vi "joystick-velout.vi"() -> (0 "error out 3":errorcluster, 2 "channel":T1)   [LabVIEW 2016]
uses:
  <extravilib>/ChannelInstances/Lossy Stream-a[.](dbl)/)Channel.ctl
  <extravilib>/ChannelInstances/Lossy Stream-a[.](dbl)/Write With Abort.vi
  <extravilib>/ChannelInstances/Lossy Stream-a[.](dbl)/Endpoint.vi
  <extravilib>/ChannelInstances/Lossy Stream-a[.](dbl)/)Channel.vi
  <resource>/ChannelSupport/_ChannelSupport/WaitIfNeeded.vi
  <vilib>/Utility/inputDevices.llb/closeJoystick.vi
  <extravilib>/ChannelInstances/Lossy Stream-a[.](dbl).lvlib
panel:
  out "16bit integer 3":i16
  out "16bit integer 2":i16
  out "16bit integer":i16
  out "appended array":u8[](array[numeric])
  in  "stop":bool
  in  "pos 1":i16=3468
  in  "pos 2":i16=3468
  in  "pos 3":i16=3468
  out "vel radial":u8[](array[numeric])
  out "vel normal":u8[](array[numeric])
  out "vel rotation":u8[](array[numeric])
  out "drible":u8
  # "vtan"
  # "vnorm"
  # "vang"
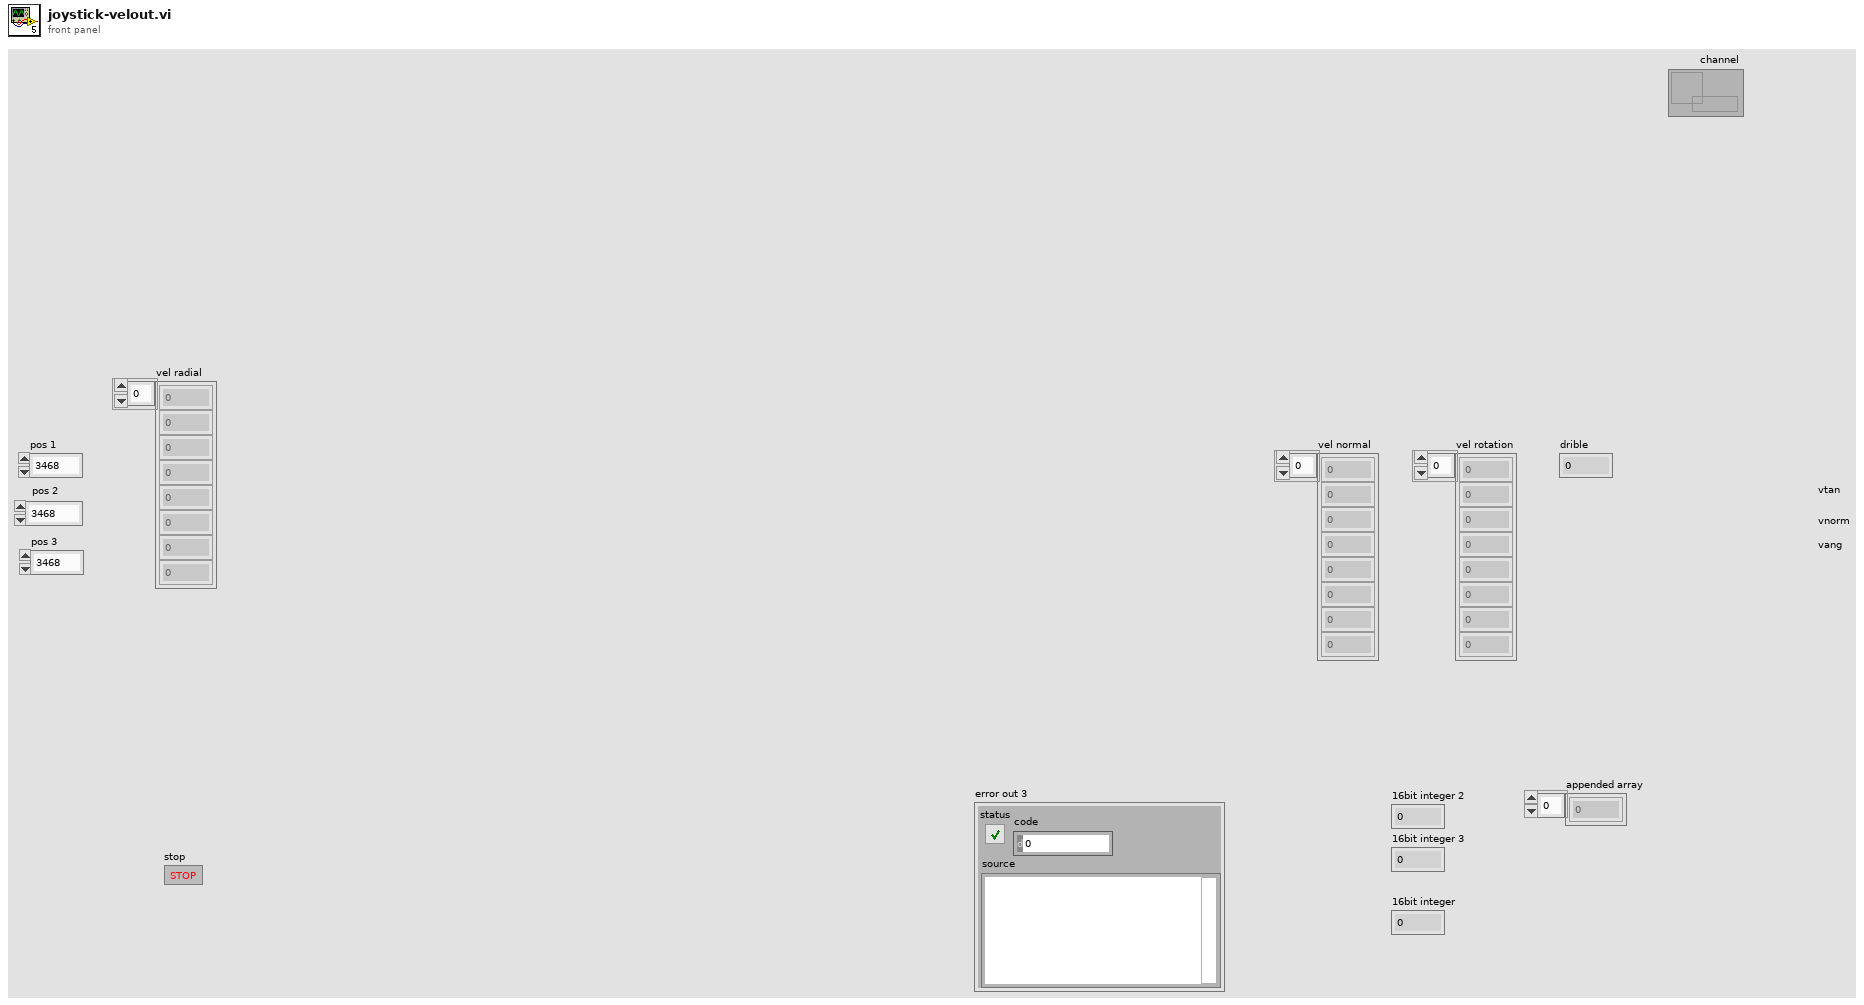
[diagram p1: front panel]
types:
  T1 = typedef "Lossy Stream-a[.](dbl).lvlib/)Channel.ctl" = refnum<queue>
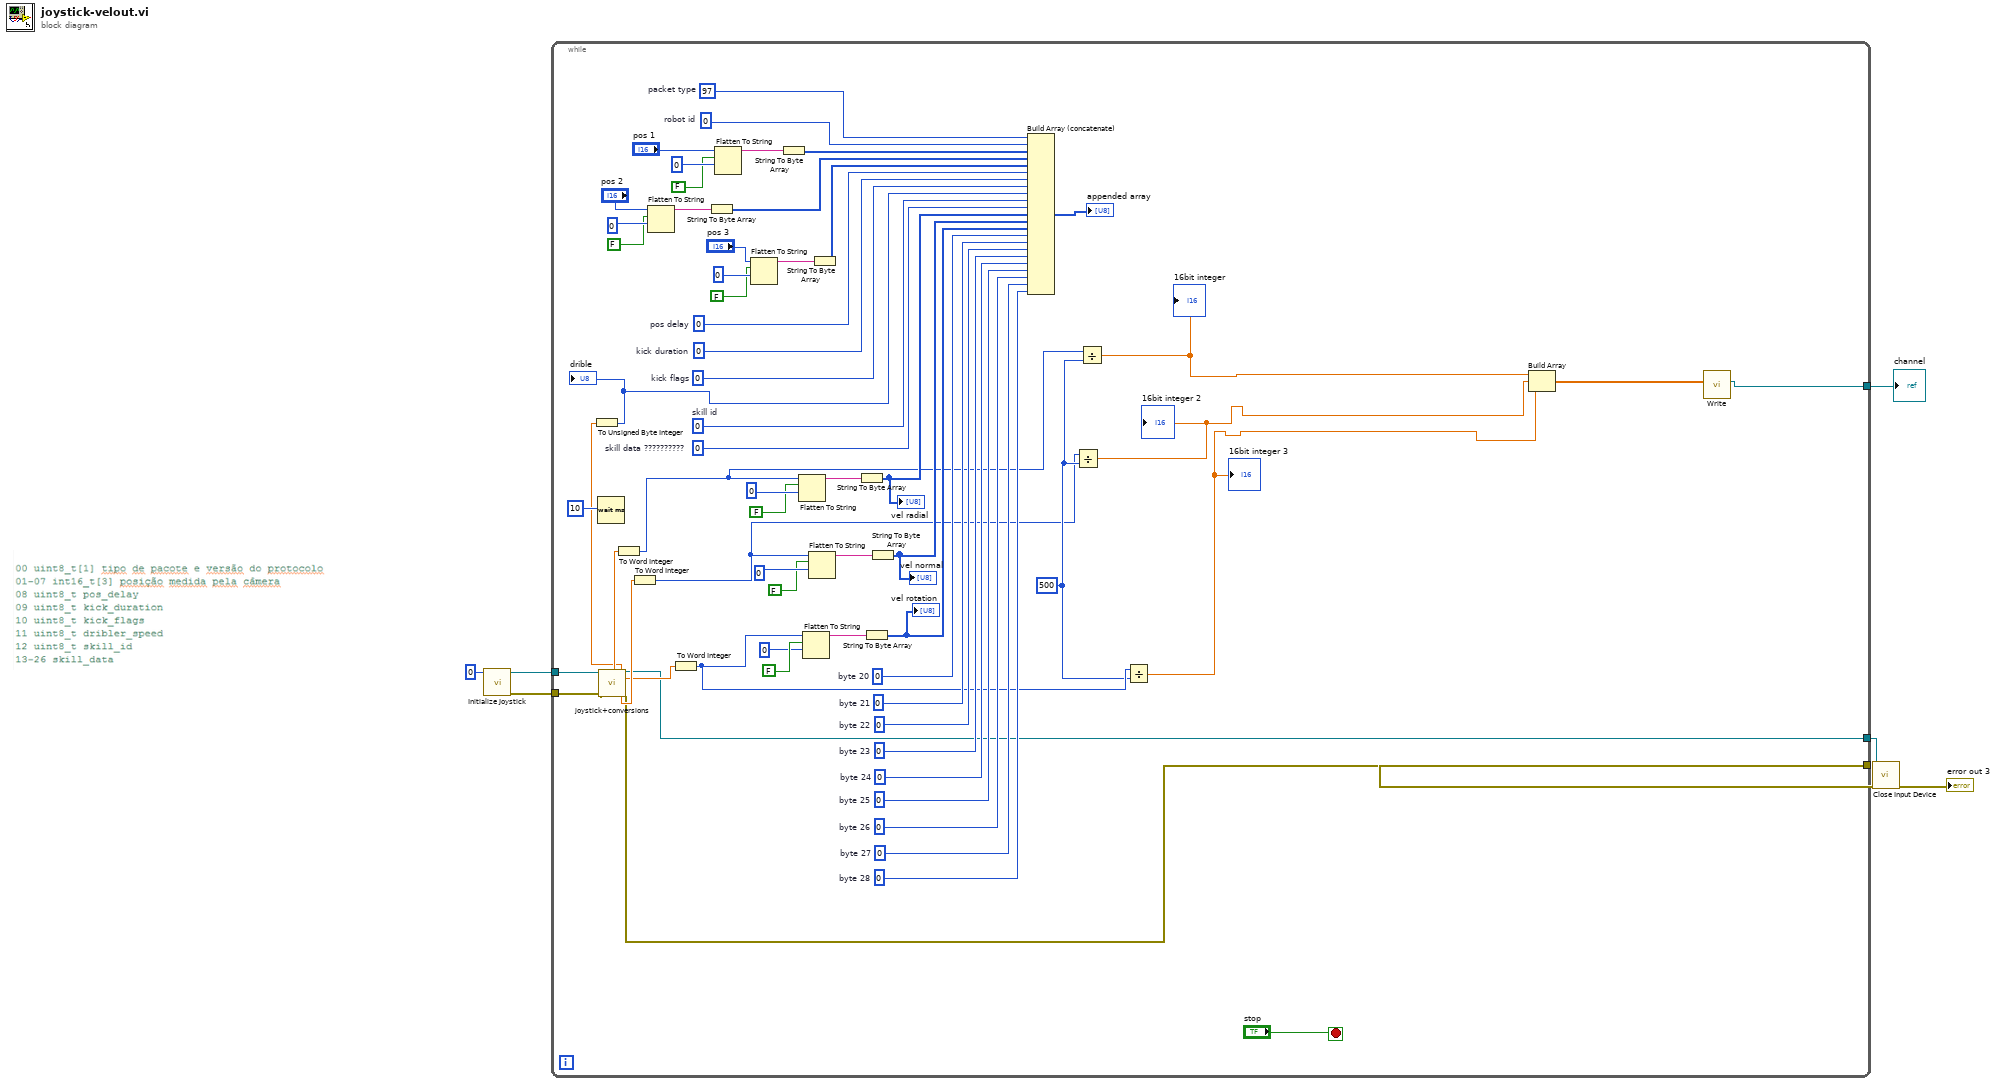
[diagram p0: block diagram]
diagram:
  n1 = call <vilib>:"Initialize Joystick.vi"("device index"=0) -> ("error out"=w5:errorcluster, "device ID"=w6:refnum<k1>)  [unwired: 9 in]
  n2 = while {
    tunnel: w6 -> [w28]
    tunnel: w5 -> [w27]
    tunnel: [w21] -> w3
    tunnel: [w20] -> w2
    tunnel: [w8] -> w1
    stop <- "stop" stop-if-true
    w14 = 500
    w70 = u8 0  # skill data ??????????
    w67 = u8 0  # byte 28
    w66 = u8 0  # byte 27
    w65 = u8 0  # byte 26
    w63 = u8 0  # byte 25
    w64 = u8 0  # byte 24
    w62 = u8 0  # byte 23
    w61 = u8 0  # byte 22
    w60 = u8 0  # byte 21
    w59 = u8 0  # byte 20
    w53 = u8 0  # skill id
    w58 = u8 0  # kick flags
    w52 = u8 0  # kick duration
    w51 = u8 0  # pos delay
    w56 = u8 0  # robot id
    w29 = u8 97  # packet type
    n3 = Wait (ms)(milliseconds to wait=u32 10) -> ()  [unwired: 1 out]
    n4 = call "joystick+conversions.vi"("Refnum in"=w28, "error in (no error)"=w27) -> ("v_radial"=w26:dbl, "drible"=w22:dbl, "v_normal"=w25:dbl, "Refnum out"=w20:refnum<k1>, "R*w"=w24:dbl, "error out"=w21:errorcluster)  [unwired: 9 in, 11 out]
    n5 = To Unsigned Byte Integer(number=w22) -> (unsigned 8bit integer=w23:u8)
    "drible" <- w23
    n6 = To Word Integer(number=w26) -> (16bit integer=w16:i16)
    n7 = To Word Integer(number=w25) -> (16bit integer=w13:i16)
    n8 = Flatten To String(anything="pos 2", prepend array or string size? (T)=FALSE, byte order (0:big-endian, network order)=u16 0) -> (data string=w37:string)  [unwired: 1 in, 2 out]
    n9 = To Word Integer(number=w24) -> (16bit integer=w15:i16)
    n10 = String To Byte Array(string=w37) -> (unsigned byte array=w57:u8[])
    n11 = Flatten To String(anything="pos 1", prepend array or string size? (T)=FALSE, byte order (0:big-endian, network order)=u16 0) -> (data string=w32:string)  [unwired: 1 in, 2 out]
    n12 = Flatten To String(anything="pos 3", prepend array or string size? (T)=FALSE, byte order (0:big-endian, network order)=u16 0) -> (data string=w41:string)  [unwired: 1 in, 2 out]
    n13 = String To Byte Array(string=w32) -> (unsigned byte array=w33:u8[])
    n14 = Flatten To String(anything=w16, prepend array or string size? (T)=FALSE, byte order (0:big-endian, network order)=u16 0) -> (data string=w46:string)  [unwired: 1 in, 2 out]
    n15 = Flatten To String(anything=w15, prepend array or string size? (T)=FALSE, byte order (0:big-endian, network order)=u16 0) -> (data string=w50:string)  [unwired: 1 in, 2 out]
    n16 = Flatten To String(anything=w13, prepend array or string size? (T)=FALSE, byte order (0:big-endian, network order)=u16 0) -> (data string=w49:string)  [unwired: 1 in, 2 out]
    n17 = String To Byte Array(string=w41) -> (unsigned byte array=w43:u8[])
    n18 = String To Byte Array(string=w46) -> (unsigned byte array=w68:u8[])
    "vel radial" <- w68
    n19 = String To Byte Array(string=w50) -> (unsigned byte array=w69:u8[])
    "vel rotation" <- w69
    n20 = String To Byte Array(string=w49) -> (unsigned byte array=w17:u8[])
    "vel normal" <- w17
    n21 = Build Array (concatenate)(w29, w56, w33, w57, w43, w51, w52, w58, w23, w53, w70, w68, w17, w69, w59, w60, w61, w62, w64, w63, w65, w66, w67) -> (→"appended array":u8[])
    n22 = Divide(x=w13, y=w14) -> (x/y=w11:dbl)
    "16bit integer 2" <- w11
    n23 = Divide(x=w16, y=w14) -> (x/y=w12:dbl)
    "16bit integer" <- w12
    n24 = Divide(x=w15, y=w14) -> (x/y=w10:dbl)
    "16bit integer 3" <- w10
    n25 = Build Array(w12, w11, w10) -> (w9:dbl[])
    n26 = call <extravilib>:"Write.vi"("element"=w9) -> ("channel"=w8:T1)  [unwired: 8 in, 2 out]
  }
  "channel" <- w1
  n27 = call-poly <vilib>:"Close Input Device.vi"("error in (no error)"=w3, "device ID"=w2) -> ("error out"=→"error out 3":errorcluster)  [unwired: 8 in]
